vi "Write Sponsor.vi"(8 "error in (no error)":errorcluster, 10 "Sponsor":string, 11 "Sports Player in":refnum<class "Sports Player.lvclass">) -> (0 "error out":errorcluster, 3 "Sports Player out":refnum<class "Sports Player.lvclass">)   [LabVIEW 2019, in "Sports Player.lvclass"]
uses:
  Sports Player.lvclass
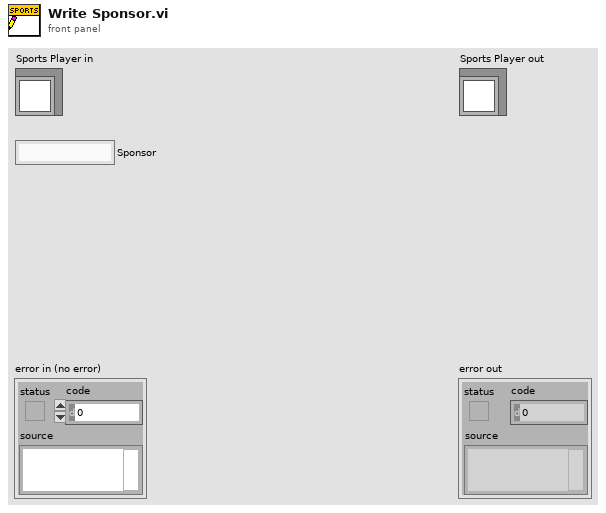
[diagram p1: front panel]
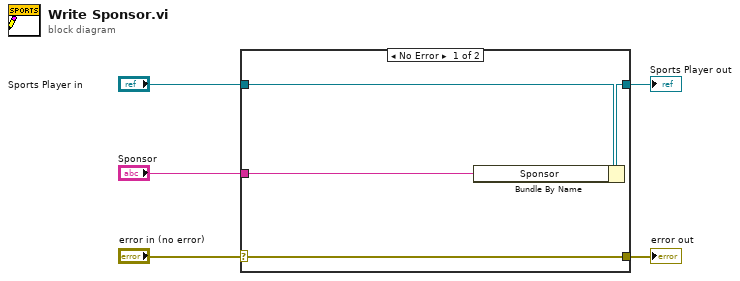
[diagram p0: block diagram]
diagram:
  n1 = case shown="No Error" "error in (no error)" {
    selector: "error in (no error)" -> [w9 w10]
    tunnel: [w9 w10] -> w4
    tunnel: [w7 w11] -> w2
    tunnel: "Sports Player in" -> [w8 w11]
    tunnel: "Sponsor" -> [w6 _]
    frame No Error {
      n2 = Bundle By Name(cluster=w8, "Sponsor"=w6) -> (w7:refnum<class "Sports Player.lvclass">)
    }
    frame Error {
    }
  }
  "error out" <- w4
  "Sports Player out" <- w2
